vi "Write Grant Flow.vi"(8 "error in (no error)":errorcluster, 10 "Grant Flow":T1=enum."Authorization Code (PKCE)", 11 "Oauth2 in":refnum<class "Oauth2.lvclass">) -> (0 "error out":errorcluster, 3 "Oauth2 out":refnum<class "Oauth2.lvclass">)   [LabVIEW 2017, in "Oauth2.lvclass"]
uses:
  Oauth2.lvclass
  OAuth2 Flow -- enum.ctl
  OAuth2 Grant Type -- ring.ctl
  LabVIEW/Oauth2/source/Oauth2/OAuth2 Response Type -- ring.ctl
  OAuthToken/OAuth2 Token Element -- enum.ctl
  Oauth2.lvclass/Oauth2.ctl
  OAuthToken/OAuthAccessToken.lvclass
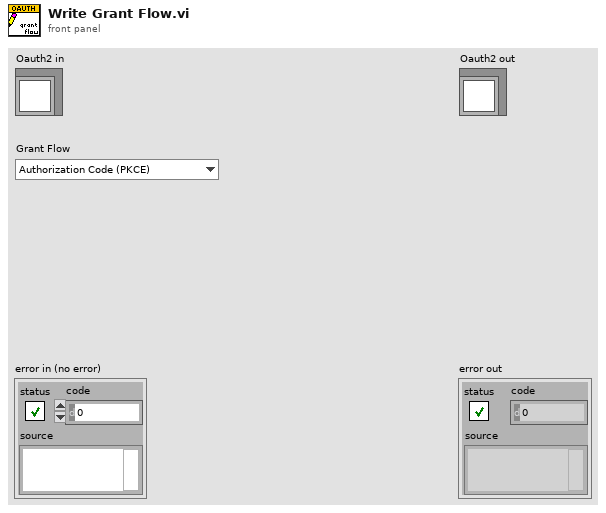
[diagram p1: front panel]
types:
  T1 = typedef "Oauth2.lvclass/OAuth2 Flow -- enum.ctl" = enum16{"Authorization Code", "Authorization Code (PKCE)", "Implicit", "Resource Owner Credentials", "Client Credentials"}
  T2 = typedef "Oauth2.lvclass/OAuth2 Response Type -- ring.ctl" = string
  T3 = typedef "Oauth2.lvclass/OAuth2 Grant Type -- ring.ctl" = string
  T4 = typedef "OAuthAccessToken.lvclass/OAuth2 Token Element -- enum.ctl" = enum16{"client_id", "client_secret", "response_type", "scope", "redirect_uri", "error", "error_description", "error_uri", "grant_type", "code", "access_token", "token_type", "expires_in", "username", "password", "refresh_token", "code_challenge", "code_challenge_method", "reverse_proxy_uri", "endpoint element", "access_type", "prompt", "id_token"}
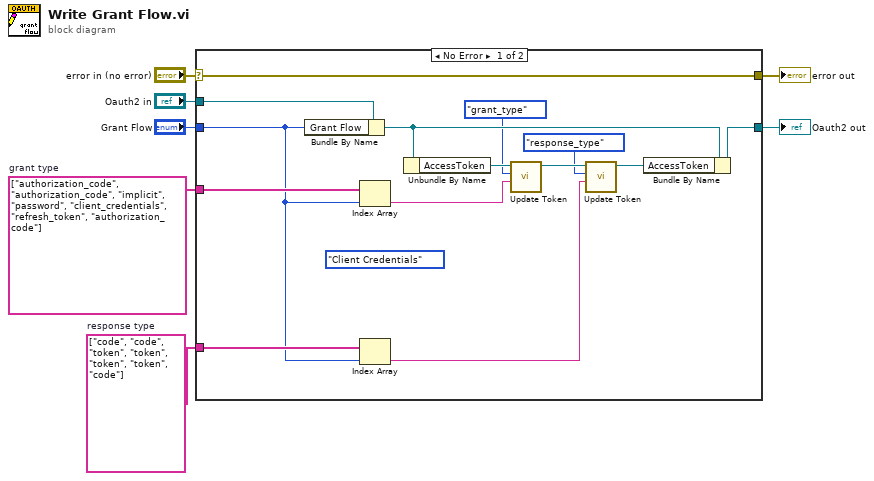
[diagram p0: block diagram]
diagram:
  w1 = T2[] ["code", "code", "token", "token", "token", "token", "code"]  # response type
  w2 = T3[] ["authorization_code", "authorization_code", "implicit", "password", "client_credentials", "refresh_token", "authorization_code"]  # grant type
  n1 = case shown="No Error" "error in (no error)" {
    selector: "error in (no error)" -> [w21 w22]
    tunnel: [w21 w22] -> w6
    tunnel: [w9 w23] -> w4
    tunnel: "Oauth2 in" -> [w20 w23]
    tunnel: "Grant Flow" -> [w11 _]
    tunnel: w2 -> [w19 _]
    tunnel: w1 -> [w12 _]
    frame No Error {
      (unwired) OAuth2_Flow_--_enum."Client Credentials" ("Grant Flow")
      n2 = Bundle By Name(cluster=w20, "Grant Flow"=w11) -> (w18:refnum<class "Oauth2.lvclass">)
      n3 = Index Array(array=w19, index=w11) -> (element=w15:T3)
      n4 = Index Array(array=w12, index=w11) -> (element=w10:T2)
      n5 = Unbundle By Name(w18) -> ("AccessToken"=w17:refnum<class "OAuthAccessToken.lvclass">)
      n6 = call "Update Token.vi"("Value"=w15, "Token element"=OAuth2_Token_Element_--_enum."grant_type", "OAuthAccessToken in"=w17) -> ("OAuthAccessToken out"=w14:refnum<class "OAuthAccessToken.lvclass">)  [unwired: 7 in, 1 out]
      n7 = call "Update Token.vi"("Value"=w10, "Token element"=OAuth2_Token_Element_--_enum."response_type", "OAuthAccessToken in"=w14) -> ("OAuthAccessToken out"=w8:refnum<class "OAuthAccessToken.lvclass">)  [unwired: 7 in, 1 out]
      n8 = Bundle By Name(cluster=w18, "AccessToken"=w8) -> (w9:refnum<class "Oauth2.lvclass">)
    }
    frame Error {
    }
  }
  "error out" <- w6
  "Oauth2 out" <- w4
